vi "Buttons Toggled.vi"(11 "Buttons":bool[](array[boolean])) -> (3 "Buttons Toggled":bool[](array[boolean]))   [LabVIEW 2019]
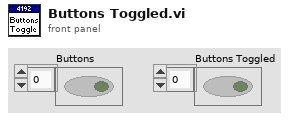
[diagram p1: front panel]
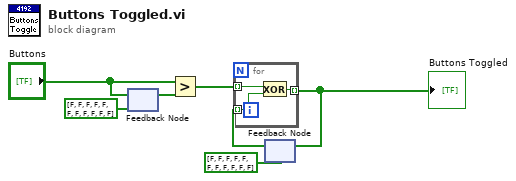
[diagram p0: block diagram]
diagram:
  n1 = feedback #1(bool[] [FALSE, FALSE, FALSE, FALSE, FALSE, FALSE, FALSE, FALSE, FALSE, FALSE, FALSE] ("Button Values")) -> (w2:bool[])
  n2 = feedback-in #1("Buttons") -> ()
  n3 = Greater?(x="Buttons", y=w2) -> (0:w7:bool[])
  n4 = feedback #2(bool[] [FALSE, FALSE, FALSE, FALSE, FALSE, FALSE, FALSE, FALSE, FALSE, FALSE, FALSE] ("Button Values")) -> (w4:bool[])
  n5 = for {
    tunnel: [w9] -> w6 mode=indexing
    tunnel: w4 -> [w10] mode=indexing
    tunnel: w7 -> [w8] mode=indexing
    n6 = Exclusive Or(1:w10, 2:w8) -> (0:w9:bool)
  }
  "Buttons Toggled" <- w6
  n7 = feedback-in #2(w6) -> ()
